vi "PDC_MRAWFileLoadOpen.vi"(0 "FileName":string, 1 "ImageBuffInfo":T1, 2 "MRawBitDepth":u32, 3 "error in (no error)":errorcluster) -> (5 "ReturnValue":u32, 6 "FileNo":u32, 7 "ErrorCode":u32, 8 "error out":errorcluster)   [LabVIEW 8.6]
doc: "This VI opens MRAW file for loading."
uses:
  PDCLIB.dll
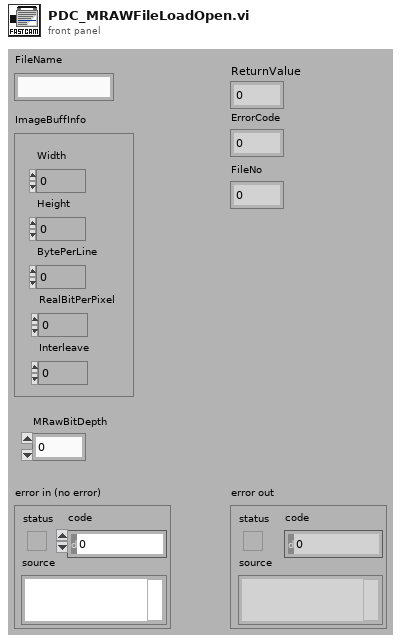
[diagram p1: front panel]
types:
  T1 = cluster{"Width":i32, "Height":i32, "BytePerLine":i32, "RealBitPerPixel":u16, "Interleave":i32}
  T2 = cluster{"Width":i32, "Height":i32, "BytePerLine":i32, "RealBitPerPixel":u16, u16, "Interleave":i32}
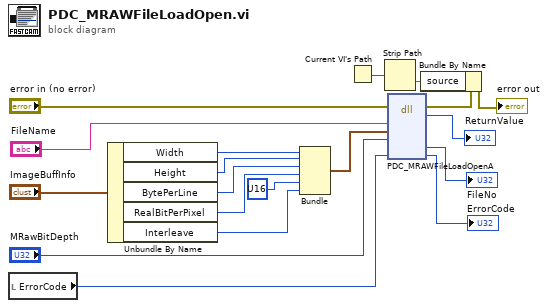
[diagram p0: block diagram]
diagram:
  n1 = local read "ErrorCode"() -> (w16:u32)
  n2 = Unbundle By Name("ImageBuffInfo") -> ("Width"=w7:i32, "Height"=w6:i32, "BytePerLine"=w4:i32, "RealBitPerPixel"=w3:u16, "Interleave"=w1:i32)
  n3 = Bundle("Width"=w7, "Height"=w6, "BytePerLine"=w4, "RealBitPerPixel"=w3, u16 ?, "Interleave"=w1) -> (w5:T2)  [unwired: 1 in]
  n4 = Current VI's Path() -> (path=w12:path)
  n5 = Strip Path(path=w12) -> (name=w13:string)  [unwired: 1 out]
  n6 = dll-call lib="PDCLIB.dll" fn="PDC_MRAWFileLoadOpenA"(error in="error in (no error)", "lpszFileName"="FileName", "pInfo"=w5, "nMRawBitDepth"="MRawBitDepth", "pErrorCode"=w16) -> (error out=w11:errorcluster, "return type"=→"ReturnValue":u32, "pFileNo"=→"FileNo":u32, "pErrorCode"=→"ErrorCode":u32)  [unwired: 6 in, 1 out]
  n7 = Bundle By Name(cluster=w11, "source"=w13) -> (→"error out":errorcluster)
